vi "message.vi"(0 "message":string="Ga on?") -> ()   [LabVIEW 2011]
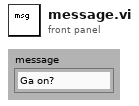
[diagram p1: front panel]
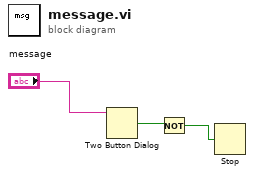
[diagram p0: block diagram]
diagram:
  n1 = Two Button Dialog(message="message") -> (T button?=w2:bool)  [unwired: 2 out]
  n2 = Not(x=w2) -> (.not. x?=w1:bool)
  n3 = Stop(stop? (T)=w1) -> ()
